vi "AB_820_850_Project_Source_Container.vi"(6 "dataForPrevious":T1, 7 "action":T6, 8 "error in (no error)":errorcluster, 9 "index in":i32, 10 "dataSource in":T5, 11 "buildObject":T4) -> (0 "error out":errorcluster, 1 "index out":i32, 2 "dataSource out":T5, 3 "buildObject out":T4)   [LabVIEW 2020]
doc: "Reads and writes the data to the object property bag."
uses:
  <resource>/Framework/Providers/API/ItemRef.ctl
  <vilib>/AppBuilder/RW_Project/AB_RW_Project_PropBag_Action.ctl
  <vilib>/AppBuilder/RW_Project/AB_RW_Project_Source_Data_for_Previous.ctl
  <vilib>/AppBuilder/AB_BuildType.ctl
  <vilib>/Utility/lvfile.llb/LVFileType.ctl
  <vilib>/Utility/lvfile.llb/NI_FileType.lvlib
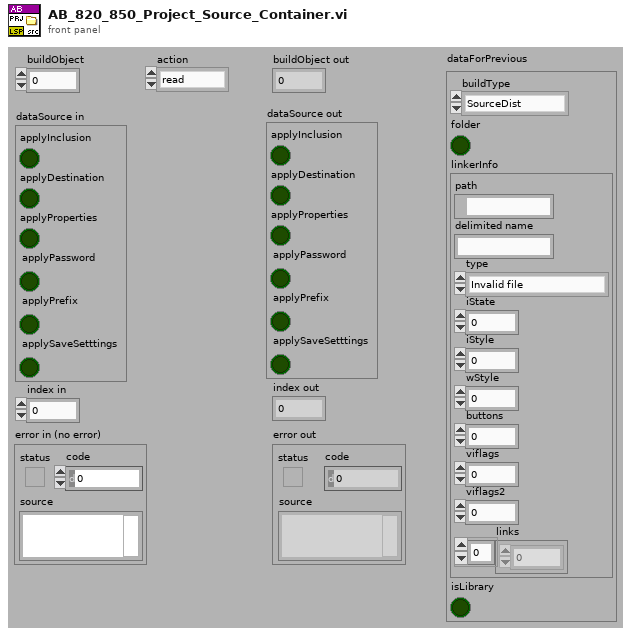
[diagram p1: front panel]
types:
  T1 = typedef "AB_RW_Project_Source_Data_for_Previous.ctl" = cluster{"buildType":T2, "folder":bool, "linkerInfo":cluster{"path":path, "delimited name":string, "type":T3, "iState":u32, "iStyle":u16, "wStyle":u16, "buttons":u16, "viflags":u32, "viflags2":u32, "links":u32[]}, "isLibrary":bool}
  T2 = typedef "AB_BuildType.ctl" = enum16{"SourceDist", "EXE", "DLL", "RTExe"}
  T3 = typedef "NI_FileType.lvlib/LVFileType.ctl" = enum32{"Invalid file", "Unknown type", "Instrument", "Control", "Polymorphic VI", "Project", "Library", "LVClass", "XControl", "XNode", "Shared library", ".NET assembly", "ActiveX interface", "CIN", "Run-time menu", "Palette menu", "Help file", "LLB", "XNode Edit Dependency", "Class Private Data Control", "Statechart", "MathScript .m file", "Ladder Diagram", "LVLibp", "XNode Build Dependency"}
  T4 = typedef "ItemRef.ctl" = u64
  T5 = cluster{"applyInclusion":bool, "applyDestination":bool, "applyProperties":bool, "applyPassword":bool, "applyPrefix":bool, "applySaveSetttings":bool}
  T6 = typedef "AB_RW_Project_PropBag_Action.ctl" = enum16{"read", "write", "clear", "readPrevious", "writePrevious", "clearPrevious"}
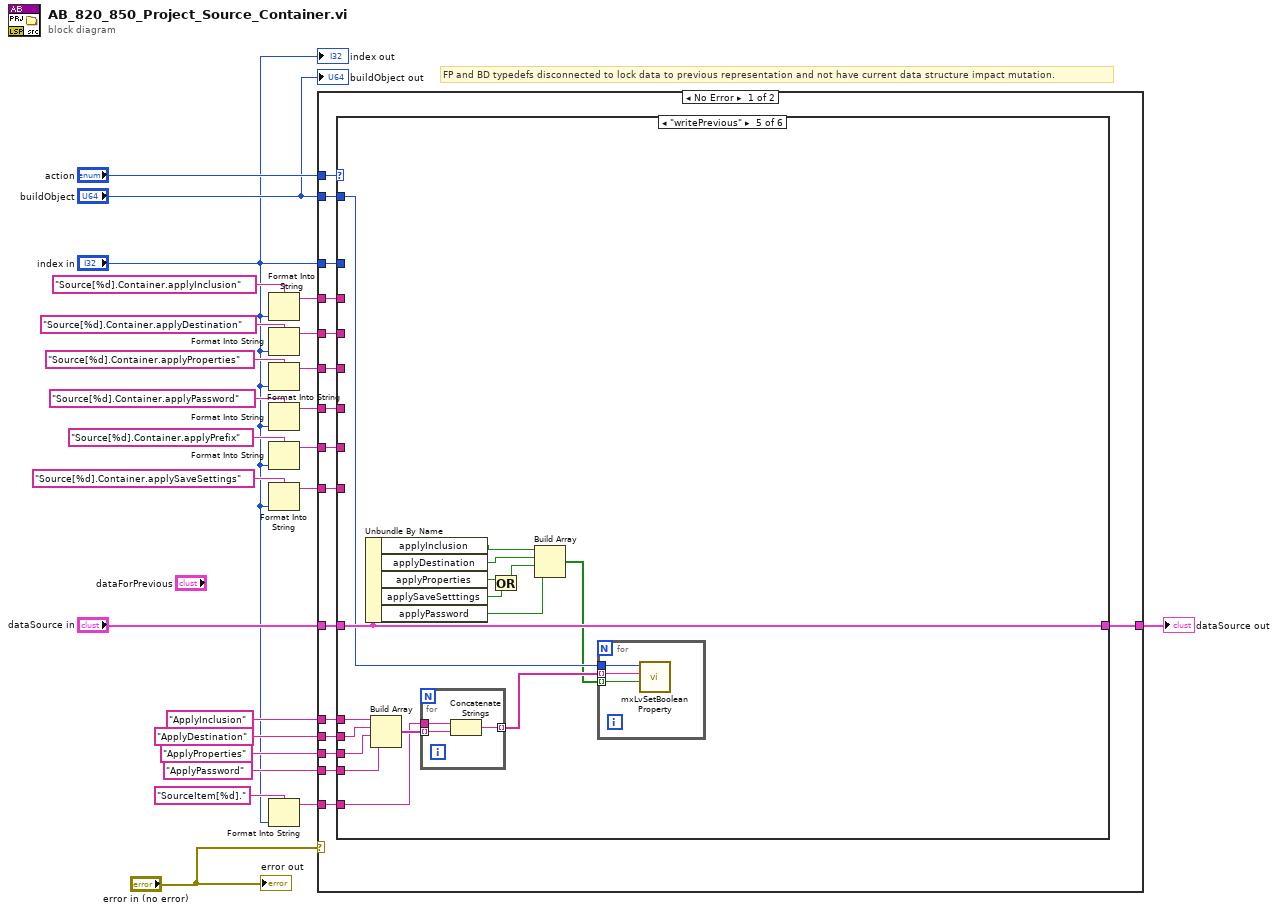
[diagram p0: block diagram]
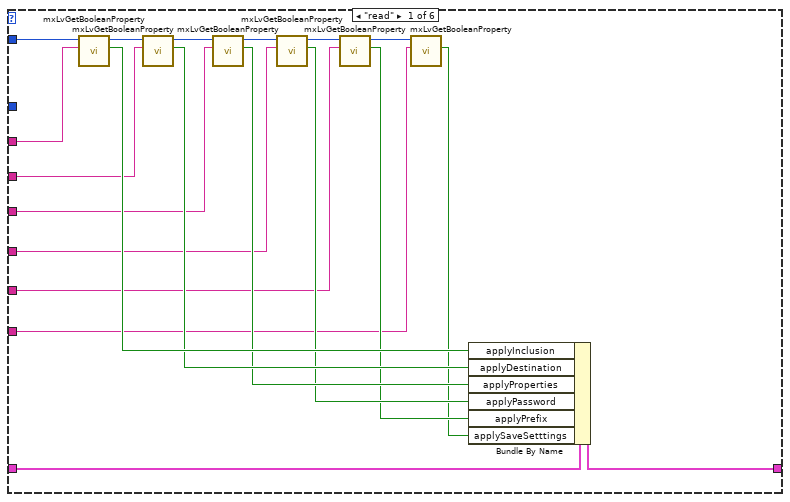
[diagram p2: hidden frame]
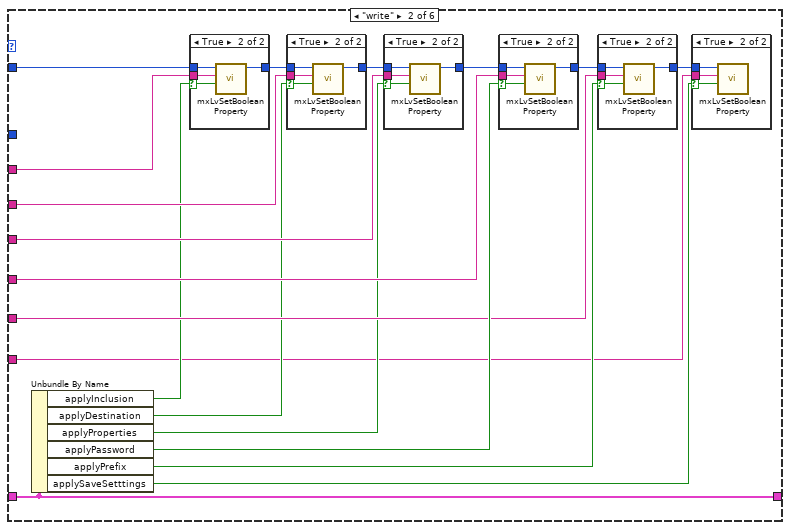
[diagram p3: hidden frame]
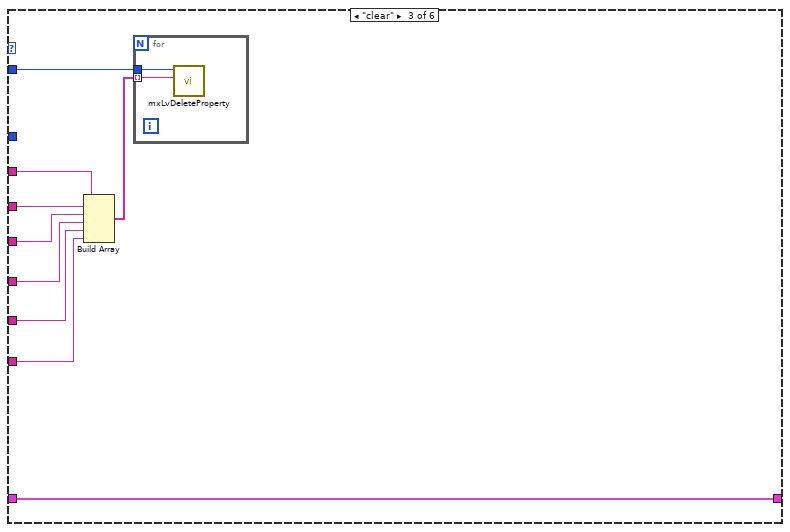
[diagram p10: hidden frame]
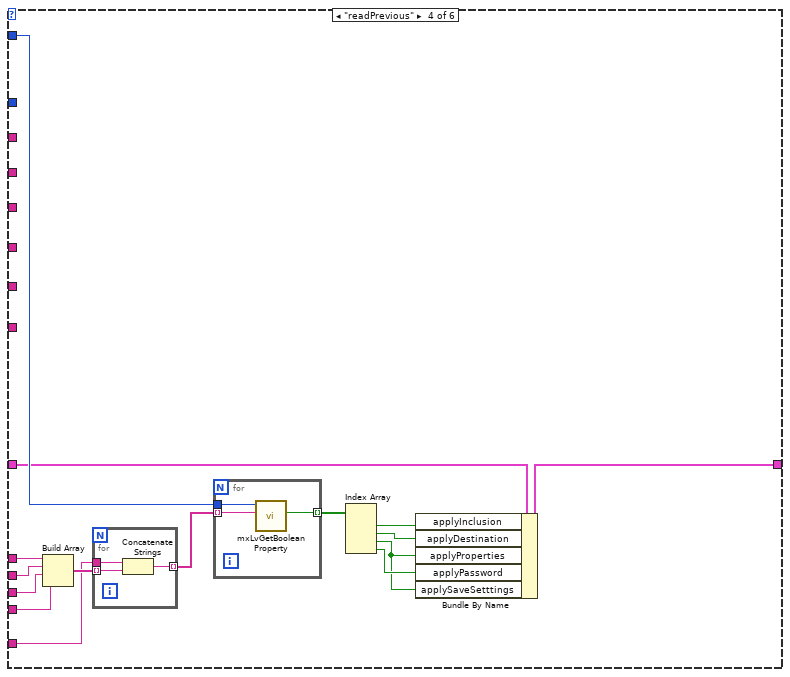
[diagram p11: hidden frame]
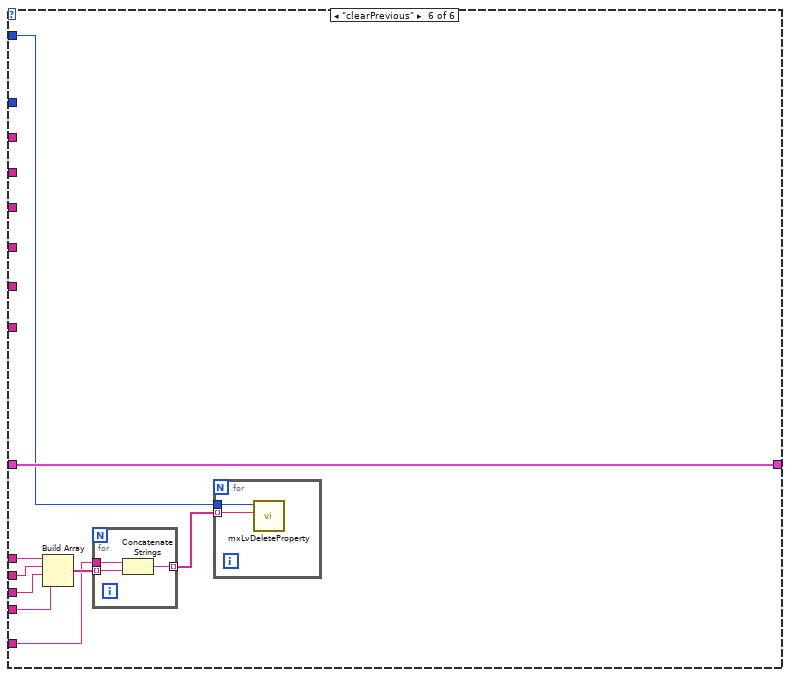
[diagram p12: hidden frame]
diagram:
  # "FP and BD typedefs disconnected to lock data to previous representation and not have current data structure impact mutation."
  n1 = Format Into String(format string="Source[%d].Container.applyInclusion", "index in") -> (resulting string=w21:string)  [unwired: 2 in, 1 out]
  n2 = Format Into String(format string="Source[%d].Container.applyDestination", "index in") -> (resulting string=w18:string)  [unwired: 2 in, 1 out]
  n3 = Format Into String(format string="Source[%d].Container.applyProperties", "index in") -> (resulting string=w17:string)  [unwired: 2 in, 1 out]
  n4 = Format Into String(format string="Source[%d].Container.applyPassword", "index in") -> (resulting string=w12:string)  [unwired: 2 in, 1 out]
  n5 = Format Into String(format string="Source[%d].Container.applyPrefix", "index in") -> (resulting string=w4:string)  [unwired: 2 in, 1 out]
  n6 = Format Into String(format string="Source[%d].Container.applySaveSettings", "index in") -> (resulting string=w1:string)  [unwired: 2 in, 1 out]
  n7 = Format Into String(format string="SourceItem[%d].", "index in") -> (resulting string=w6:string)  [unwired: 2 in, 1 out]
  n8 = case shown="No Error" "error in (no error)" {
    tunnel: "action" -> [w40 _]
    tunnel: "dataSource in" -> [w39 w176]
    tunnel: w21 -> [w38 _]
    tunnel: w18 -> [w37 _]
    tunnel: w17 -> [w36 _]
    tunnel: "index in" -> [w35 _]
    tunnel: [w34 w176] -> w16
    tunnel: "buildObject" -> [w33 _]
    tunnel: w12 -> [w32 _]
    tunnel: "ApplyInclusion" -> [w31 _]
    tunnel: "ApplyDestination" -> [w30 _]
    tunnel: "ApplyProperties" -> [w29 _]
    tunnel: "ApplyPassword" -> [w28 _]
    tunnel: w6 -> [w27 _]
    tunnel: w4 -> [w26 _]
    tunnel: w1 -> [w25 _]
    frame No Error {
      n9 = case shown="\"writePrevious\"" w40 {
        tunnel: w33 -> [w58 w76 w111 w127 w147 w162]
        tunnel: w39 -> [w60 w79 w116 w124 w155 w170]
        tunnel: w38 -> [w56 w72 w115 _ _ _]
        tunnel: w37 -> [w53 w71 w114 _ _ _]
        tunnel: w36 -> [w51 w70 w113 _ _ _]
        tunnel: w35 -> [_ _ _ _ _ _]
        tunnel: [w59 w79 w116 w123 w155 w170] -> w34
        tunnel: w32 -> [w48 w78 w110 _ _ _]
        tunnel: w31 -> [_ _ _ w133 w152 w167]
        tunnel: w30 -> [_ _ _ w132 w151 w166]
        tunnel: w29 -> [_ _ _ w131 w150 w165]
        tunnel: w28 -> [_ _ _ w130 w149 w164]
        tunnel: w27 -> [_ _ _ w128 w148 w163]
        tunnel: w26 -> [w46 w68 w109 _ _ _]
        tunnel: w25 -> [w42 w62 w108 _ _ _]
        frame "read" {
          n10 = call <resource>:"mxLvGetBooleanProperty.vi"("Tag"=w56, "Item"=w58) -> ("Value"=w57:bool, "Item"=w55:T4)  [unwired: 7 in, 1 out]
          n11 = call <resource>:"mxLvGetBooleanProperty.vi"("Tag"=w53, "Item"=w55) -> ("Value"=w52:bool, "Item"=w54:T4)  [unwired: 7 in, 1 out]
          n12 = call <resource>:"mxLvGetBooleanProperty.vi"("Tag"=w51, "Item"=w54) -> ("Value"=w50:bool, "Item"=w49:T4)  [unwired: 7 in, 1 out]
          n13 = call <resource>:"mxLvGetBooleanProperty.vi"("Tag"=w48, "Item"=w49) -> ("Value"=w47:bool, "Item"=w45:T4)  [unwired: 7 in, 1 out]
          n14 = call <resource>:"mxLvGetBooleanProperty.vi"("Tag"=w46, "Item"=w45) -> ("Value"=w43:bool, "Item"=w44:T4)  [unwired: 7 in, 1 out]
          n15 = call <resource>:"mxLvGetBooleanProperty.vi"("Tag"=w42, "Item"=w44) -> ("Value"=w41:bool)  [unwired: 7 in, 2 out]
          n16 = Bundle By Name(cluster=w60, "applyInclusion"=w57, "applyDestination"=w52, "applyProperties"=w50, "applyPassword"=w47, "applyPrefix"=w43, "applySaveSetttings"=w41) -> (w59:T5)
        }
        frame "write" {
          n17 = Unbundle By Name(w79) -> ("applyInclusion"=w67:bool, "applyDestination"=w66:bool, "applyProperties"=w65:bool, "applyPassword"=w77:bool, "applyPrefix"=w64:bool, "applySaveSetttings"=w61:bool)
          n18 = case shown="True" w67 {
            selector: w67 -> [_ w100]
            tunnel: w76 -> [w98 w102]
            tunnel: w72 -> [_ w101]
            tunnel: [w98 w99] -> w75
            frame False {
            }
            frame True {
              n19 = call <resource>:"mxLvSetBooleanProperty.vi"("Value (F)"=w100, "Tag"=w101, "Item"=w102) -> ("Item"=w99:T4)  [unwired: 7 in, 1 out]
            }
          }
          n20 = case shown="True" w66 {
            selector: w66 -> [_ w95]
            tunnel: w75 -> [w93 w97]
            tunnel: w71 -> [_ w96]
            tunnel: [w93 w94] -> w69
            frame False {
            }
            frame True {
              n21 = call <resource>:"mxLvSetBooleanProperty.vi"("Value (F)"=w95, "Tag"=w96, "Item"=w97) -> ("Item"=w94:T4)  [unwired: 7 in, 1 out]
            }
          }
          n22 = case shown="True" w65 {
            selector: w65 -> [_ w90]
            tunnel: w69 -> [w88 w92]
            tunnel: w70 -> [_ w91]
            tunnel: [w88 w89] -> w74
            frame False {
            }
            frame True {
              n23 = call <resource>:"mxLvSetBooleanProperty.vi"("Value (F)"=w90, "Tag"=w91, "Item"=w92) -> ("Item"=w89:T4)  [unwired: 7 in, 1 out]
            }
          }
          n24 = case shown="True" w77 {
            selector: w77 -> [_ w105]
            tunnel: w74 -> [w103 w107]
            tunnel: w78 -> [_ w106]
            tunnel: [w103 w104] -> w73
            frame False {
            }
            frame True {
              n25 = call <resource>:"mxLvSetBooleanProperty.vi"("Value (F)"=w105, "Tag"=w106, "Item"=w107) -> ("Item"=w104:T4)  [unwired: 7 in, 1 out]
            }
          }
          n26 = case shown="True" w64 {
            selector: w64 -> [_ w85]
            tunnel: w73 -> [w83 w87]
            tunnel: w68 -> [_ w86]
            tunnel: [w83 w84] -> w63
            frame False {
            }
            frame True {
              n27 = call <resource>:"mxLvSetBooleanProperty.vi"("Value (F)"=w85, "Tag"=w86, "Item"=w87) -> ("Item"=w84:T4)  [unwired: 7 in, 1 out]
            }
          }
          n28 = case shown="True" w61 {
            selector: w61 -> [_ w80]
            tunnel: w63 -> [_ w82]
            tunnel: w62 -> [_ w81]
            frame False {
            }
            frame True {
              n29 = call <resource>:"mxLvSetBooleanProperty.vi"("Value (F)"=w80, "Tag"=w81, "Item"=w82) -> ()  [unwired: 7 in, 2 out]
            }
          }
        }
        frame "clear" {
          n30 = Build Array(w115, w114, w113, w110, w109, w108) -> (w112:string[])
          n31 = for {
            tunnel: w111 -> [w118]
            tunnel: w112 -> [w117] mode=indexing
            n32 = call <resource>:"mxLvDeleteProperty.vi"("Tag"=w117, "Item"=w118) -> ()  [unwired: 8 in, 2 out]
          }
        }
        frame "readPrevious" {
          n33 = Build Array(w133, w132, w131, w130) -> (w129:string[])
          n34 = for {
            tunnel: w129 -> [w139] mode=indexing
            tunnel: w128 -> [w138]
            tunnel: [w137] -> w126 mode=indexing
            n35 = Concatenate Strings(w138, w139) -> (w137:string)
          }
          n36 = for {
            tunnel: w127 -> [w136]
            tunnel: w126 -> [w135] mode=indexing
            tunnel: [w134] -> w125 mode=indexing
            n37 = call <resource>:"mxLvGetBooleanProperty.vi"("Tag"=w135, "Item"=w136) -> ("Value"=w134:bool)  [unwired: 7 in, 2 out]
          }
          n38 = Index Array(array=w125) -> (element #1=w122:bool, element #2=w121:bool, element #3=w119:bool, element #4=w120:bool)  [unwired: 4 in]
          n39 = Bundle By Name(cluster=w124, "applyInclusion"=w122, "applyDestination"=w121, "applyProperties"=w119, "applyPassword"=w120, "applySaveSetttings"=w119) -> (w123:T5)
        }
        frame "writePrevious" {
          n40 = Unbundle By Name(w155) -> ("applyInclusion"=w146:bool, "applyDestination"=w145:bool, "applyProperties"=w141:bool, "applySaveSetttings"=w142:bool, "applyPassword"=w144:bool)
          n41 = Build Array(w152, w151, w150, w149) -> (w154:string[])
          n42 = for {
            tunnel: w154 -> [w161] mode=indexing
            tunnel: w148 -> [w160]
            tunnel: [w159] -> w153 mode=indexing
            n43 = Concatenate Strings(w160, w161) -> (w159:string)
          }
          n44 = Or(x=w141, y=w142) -> (x .or. y?=w140:bool)
          n45 = Build Array(w146, w145, w140, w144) -> (w143:bool[])
          n46 = for {
            tunnel: w147 -> [w158]
            tunnel: w153 -> [w157] mode=indexing
            tunnel: w143 -> [w156] mode=indexing
            n47 = call <resource>:"mxLvSetBooleanProperty.vi"("Value (F)"=w156, "Tag"=w157, "Item"=w158) -> ()  [unwired: 7 in, 2 out]
          }
        }
        frame "clearPrevious" {
          n48 = Build Array(w167, w166, w165, w164) -> (w169:string[])
          n49 = for {
            tunnel: w169 -> [w175] mode=indexing
            tunnel: w163 -> [w174]
            tunnel: [w173] -> w168 mode=indexing
            n50 = Concatenate Strings(w174, w175) -> (w173:string)
          }
          n51 = for {
            tunnel: w162 -> [w172]
            tunnel: w168 -> [w171] mode=indexing
            n52 = call <resource>:"mxLvDeleteProperty.vi"("Tag"=w171, "Item"=w172) -> ()  [unwired: 8 in, 2 out]
          }
        }
      }
    }
    frame Error {
    }
  }
  "dataSource out" <- w16
  "error out" <- "error in (no error)"
  "buildObject out" <- "buildObject"
  "index out" <- "index in"
